vi "Get Node Reference.vi"(8 "error in":errorcluster, 11 "Item Ref in":u64 format="%.0x") -> (0 "error out":errorcluster, 1 "Base Node":refnum<k24>, 2 "Base Node Type":refnum<k24>, 3 "Item Ref out":u64 format="%.0x")   [LabVIEW 2026, in "NIDMM Configuration.lvlib"]
uses:
  NIDMM Configuration.lvlib
  NationalInstruments.VeriStand.SystemStorage
  NationalInstruments.VeriStand.SystemDefinitionAPI
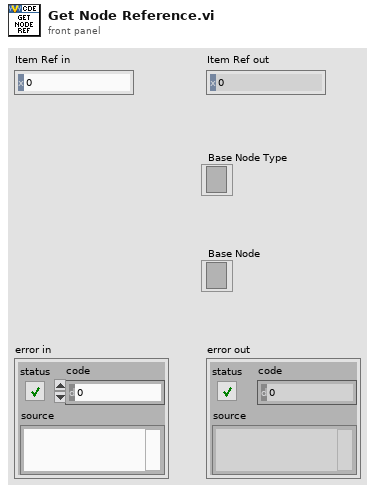
[diagram p1: front panel]
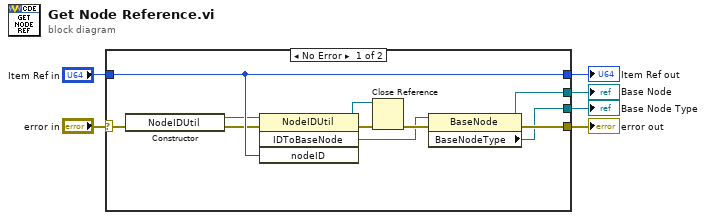
[diagram p0: block diagram]
diagram:
  n1 = case shown="No Error" "error in" {
    selector: "error in" -> [w17 w19]
    tunnel: [w16 w19] -> w5
    tunnel: [w15 _] -> w4
    tunnel: "Item Ref in" -> [w14 w18]
    tunnel: [w14 w18] -> w2
    tunnel: [w7 _] -> w1
    frame No Error {
      n2 = constructor class="NodeIDUtil"(error in=w17) -> (reference out=w9:refnum<k24>, error out=w11:errorcluster)  [unwired: 2 in, 1 out]
      n3 = invoke class="NodeIDUtil" method="IDToBaseNode"(reference=w9, error in=w11, "nodeID"=w14) -> (reference out=w10:refnum<k24>, error out=w12:errorcluster, "IDToBaseNode"=w8:refnum<k24>)  [unwired: 1 in, 1 out]
      n4 = Close Reference(reference=w10, error in (no error)=w12) -> (error out=w13:errorcluster)
      n5 = property class="BaseNode"(reference=w8, error in=w13) -> (reference out=w7:refnum<k24>, error out=w16:errorcluster, "BaseNodeType"=w15:refnum<k24>)
    }
    frame Error {
    }
  }
  "error out" <- w5
  "Base Node Type" <- w4
  "Item Ref out" <- w2
  "Base Node" <- w1
